vi "Init.vi"(0 "ActionBeep in":refnum<class "ActionBeep.lvclass">, 1 "IniFile":path, 5 "error in (no error)":errorcluster) -> (14 "ActionBeep out":refnum<class "ActionBeep.lvclass">, 19 "error out":errorcluster)   [LabVIEW 2017, in "ActionBeep.lvclass"]
doc: "Base class implementation (empty)."
uses:
  ActionBeep.lvclass
  <vilib>/Waveform/WDTOps.llb/WDT Append Waveforms DBL.vi
  <vilib>/measure/NI_MABase.lvlib
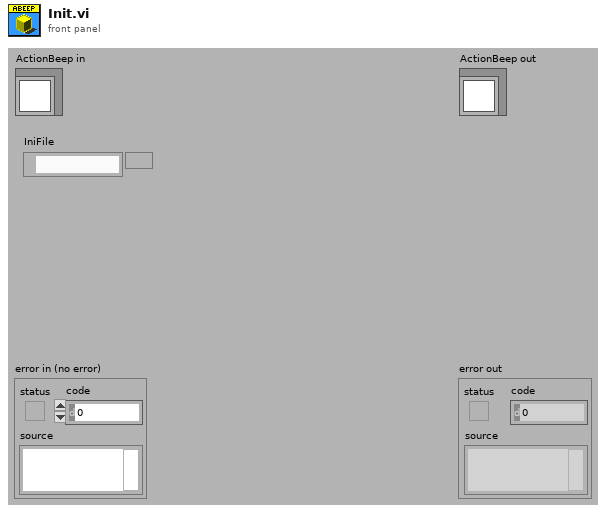
[diagram p1: front panel]
types:
  T1 = enum16{"Sine Wave", "Triangle Wave", "Square Wave", "Sawtooth Wave"}
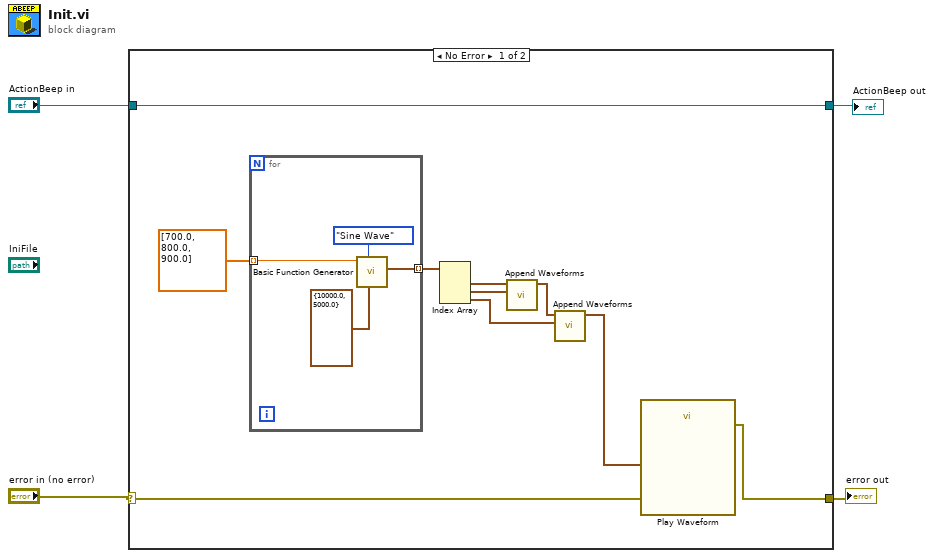
[diagram p0: block diagram]
diagram:
  n1 = case shown="No Error" "error in (no error)" {
    selector: "error in (no error)" -> [w13 w19]
    tunnel: "ActionBeep in" -> [w14 w20]
    tunnel: [w14 w20] -> w2
    tunnel: [w12 w19] -> w1
    frame No Error {
      n2 = for {
        tunnel: [w16] -> w10 mode=indexing
        tunnel: dbl[] [700.0, 800.0, 900.0] -> [w15] mode=indexing
        n3 = call <vilib>:"Basic Function Generator.vi"("sampling info"=cluster{"Fs":dbl, "#s":dbl} {"Fs"=10000.0, "#s"=5000.0}, "signal type"=T1."Sine Wave", "frequency"=w15) -> ("signal out"=w16:waveform(dbl))  [unwired: 6 in, 2 out]
      }
      n4 = Index Array(array=w10) -> (element #1=w9:waveform(dbl), element #2=w8:waveform(dbl), element #3=w6:waveform(dbl))  [unwired: 3 in]
      n5 = call-poly <vilib>:"Append Waveforms.vi"("waveform B"=w8, "waveform A"=w9) -> ("waveform out"=w7:waveform(dbl))  [unwired: 8 in, 1 out]
      n6 = call-poly <vilib>:"Append Waveforms.vi"("waveform B"=w6, "waveform A"=w7) -> ("waveform out"=w5:waveform(dbl))  [unwired: 8 in, 1 out]
      n7 = call "Play Waveform"("Data"=w5, "error in"=w13) -> ("error out"=w12:errorcluster)  [unwired: 17 in]
    }
    frame Error {
    }
  }
  "error out" <- w1
  "ActionBeep out" <- w2
